vi "dfd_Nyquist Filter Design Build Nyquist by Window.vi"(1 "FFT size":i32, 2 "window length":i32) -> (0 "nyquist filter spectrum":dbl[](array[numeric]))   [LabVIEW 2017, in "NI_DigFilter_Process.lvlib"]
uses:
  <vilib>/addons/Digital Filter Design/NI_DigFilter_Process.lvlib
  <vilib>/Analysis/4window.llb/Hanning Window (DBL).vi
  <vilib>/Analysis/4window.llb/AllCosWindow (DBL).vi
  <vilib>/Analysis/NI_AALPro.lvlib
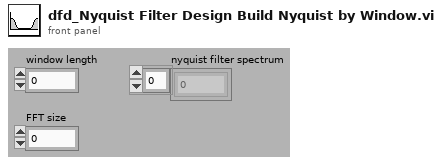
[diagram p1: front panel]
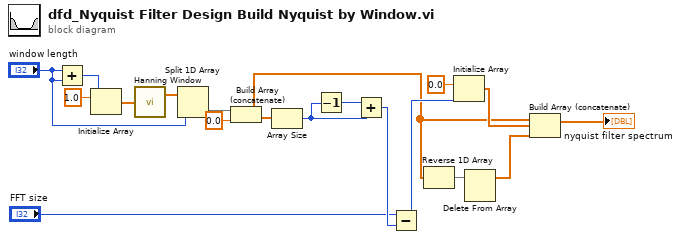
[diagram p0: block diagram]
diagram:
  n1 = Add(x="window length", y="window length") -> (x+y=w5:i32)
  n2 = Initialize Array(1.0 ("element"), w5) -> (w8:dbl[])
  n3 = call-poly <vilib>:"Hanning Window.vi"("X"=w8) -> ("Windowed X"=w7:dbl[])  [unwired: 1 out]
  n4 = Split 1D Array(array=w7, index="window length") -> (second subarray=w3:dbl[])  [unwired: 1 out]
  n5 = Build Array (concatenate)(w3, 0.0 ("element")) -> (w1:dbl[])
  n6 = Array Size(array=w1) -> (size(s)=w16:i32)
  n7 = Decrement(x=w16) -> (x-1=w15:i32)
  n8 = Add(x=w15, y=w16) -> (x+y=w13:i32)
  n9 = Subtract(x="FFT size", y=w13) -> (x-y=w14:i32)
  n10 = Reverse 1D Array(array=w1) -> (reversed array=w12:dbl[])
  n11 = Initialize Array(0.0 ("element"), w14) -> (w11:dbl[])
  n12 = Delete From Array(array=w12) -> (array with subset deleted=w2:dbl[])  [unwired: 2 in, 1 out]
  n13 = Build Array (concatenate)(w1, w11, w2) -> (→"nyquist filter spectrum":dbl[])
